vi "NonzeroArray.vi"(0 "Input Array":dbl[](array[numeric])=[1.0, 2.0, 3.0, 4.0]) -> (1 "Output Array":dbl[](array[numeric]))   [LabVIEW 2013]
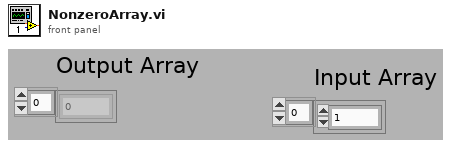
[diagram p1: front panel]
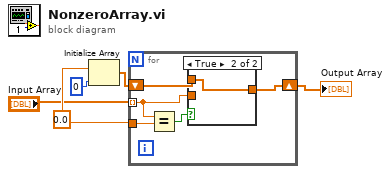
[diagram p0: block diagram]
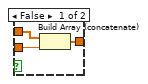
[diagram p2: hidden frame]
diagram:
  w3 = 0.0
  n1 = Initialize Array(w3, 0) -> (w4:dbl[])
  n2 = for {
    shift-right: [w7] -> w1
    shift-left: w4 -> [w8]
    tunnel: w3 -> [w10]
    tunnel: "Input Array" -> [w6] mode=indexing
    n3 = Equal?(x=w6, y=w10) -> (x = y?=w9:bool)
    n4 = case shown="True" w9 {
      tunnel: w8 -> [w11 w14]
      tunnel: [w13 w14] -> w7
      tunnel: w6 -> [w12 _]
      frame False {
        n5 = Build Array (concatenate)(w11, w12) -> (w13:dbl[])
      }
      frame True {
      }
    }
  }
  "Output Array" <- w1
